vi "Is Zombie.vi"(8 "Error In":errorcluster) -> (0 "Error Out":errorcluster)   [LabVIEW 2017, in "Tests.lvlib" / "Toolkit.lvlib"]
uses:
  Toolkit/Toolkit.lvlib
  <vilib>/Utility/traverseref.llb/TRef TravTarget.ctl
  <vilib>/addons/_JKI Toolkits/Caraya/classes/Test/Test.lvclass
  <vilib>/addons/_JKI Toolkits/Caraya/classes/Assert/Assert.lvclass
  <vilib>/Utility/traverseref.llb/VI Scripting - Traverse.lvlib
  src/Toolkit/Toolkit.lvlib
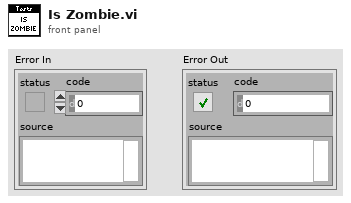
[diagram p1: front panel]
types:
  T1 = typedef "TRef TravTarget.ctl" = enum16{"FP", "BD", "Other"}
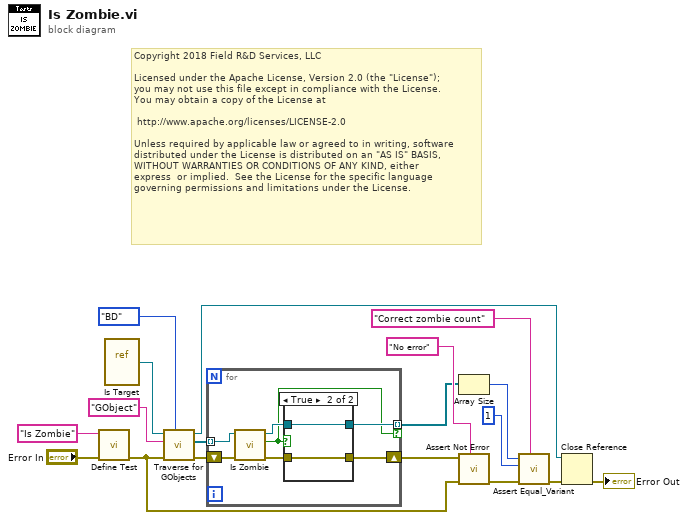
[diagram p0: block diagram]
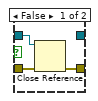
[diagram p2: hidden frame]
diagram:
  # "Copyright 2018 Field R&D Services, LLC\n\nLicensed under the Apache License, Version 2.0 (the \"License\");\nyou may not use this file except in compliance with the License.\nYou may obtain a copy of the License at\n\n\thttp://www.apache.org/licenses/LICENSE-2.0\n\nUnless required by applicable law or agreed to in writing, software\ndistributed under the License is distributed on an \"AS IS\" BASIS,\nWITHOUT WARRANTIES OR CONDITIONS OF ANY KIND, either \nexpress  or implied.  See the License for the specific language \ngoverning permissions and limitations under the License."
  n1 = call <vilib>:"Define Test.vi"("error in (no error)"="Error In", "Label (VI Title)"="Is Zombie") -> ("error out"=w9:errorcluster)  [unwired: 9 in]
  n2 = vi-ref "Is Target.vi"() -> (w7:refnum<vi>)
  n3 = call <vilib>:"Traverse for GObjects.vi"("Traverse Target"=TRef_TravTarget."BD", "error in (no error)"=w9, "Class Name"="GObject", "VI Refnum"=w7) -> ("error out"=w8:errorcluster, "References"=w6:refnum<vi>[], "dup VI Refnum"=w2:refnum<vi>)  [unwired: 4 in, 1 out]
  n4 = for {
    shift-right: [w19] -> w18
    shift-left: w8 -> [w25]
    tunnel: w6 -> [w24] mode=indexing
    tunnel: [w22] -> w4 mode=indexing if=w21
    n5 = call "Is Zombie.vi"("Error In"=w25, "GObject In"=w24) -> ("Error Out"=w20:errorcluster, "Zombie?"=w21:bool, "GObject Out"=w23:refnum<vi>)  [unwired: 7 in]
    n6 = case shown="True" w21 {
      tunnel: w23 -> [w28 w30]
      tunnel: [_ w30] -> w22
      tunnel: w20 -> [w27 w29]
      tunnel: [w26 w29] -> w19
      frame False {
        n7 = Close Reference(reference=w28, error in (no error)=w27) -> (error out=w26:errorcluster)
      }
      frame True {
      }
    }
  }
  n8 = Array Size(array=w4) -> (size(s)=w11:i32)
  n9 = call <vilib>:"Assert Not Error.vi"("Label"="No error", "error in (no error)"=w9, "Not Error?"=w18) -> ("error out"=w15:errorcluster)  [unwired: 8 in]
  n10 = call <vilib>:"Assert Equal_Variant.vi"("Label"="Correct zombie count", "error in (no error)"=w15, "Y"=1 ("size(s)"), "X"=w11) -> ("error out"=w12:errorcluster)  [unwired: 7 in]
  n11 = Close Reference(reference=w2, error in (no error)=w12) -> (error out=→"Error Out":errorcluster)
